vi "Left and Right Parts.vi"(0 "after":string, 1 "before":string) -> (2 "left start":string, 3 "left end":string, 4 "right start":string, 5 "right end":string)   [LabVIEW 2017, in "NI_Gmath.lvlib"]
uses:
  <vilib>/gmath/NI_Gmath.lvlib
panel:
  # "`"
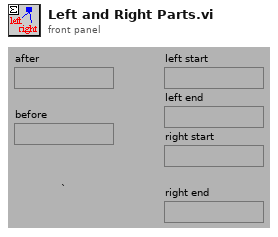
[diagram p1: front panel]
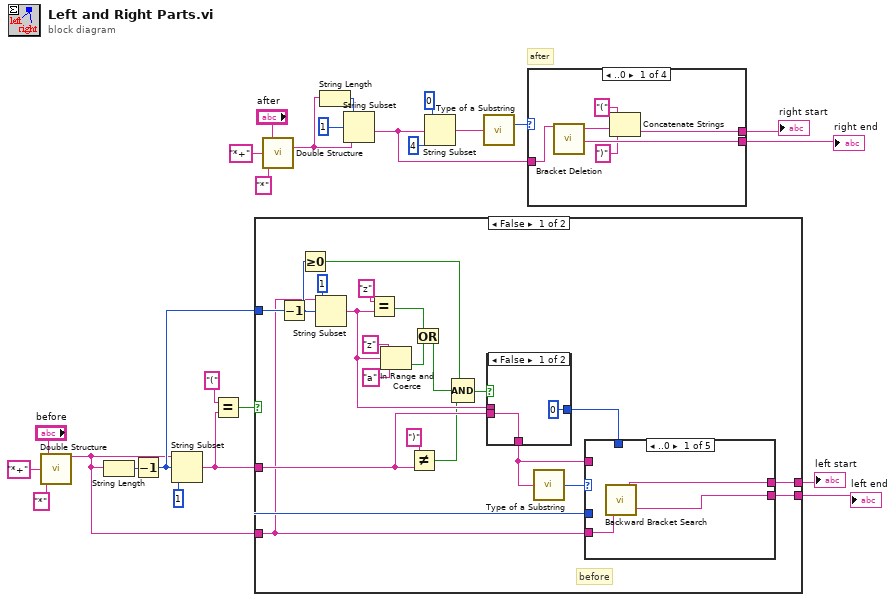
[diagram p0: block diagram]
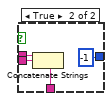
[diagram p2: hidden frame]
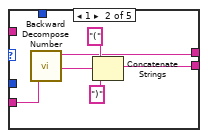
[diagram p3: hidden frame]
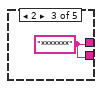
[diagram p4: hidden frame]
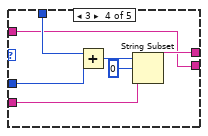
[diagram p5: hidden frame]
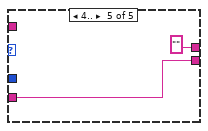
[diagram p6: hidden frame]
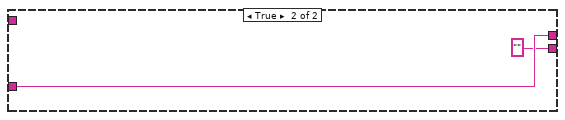
[diagram p7: hidden frame]
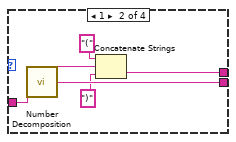
[diagram p8: hidden frame]
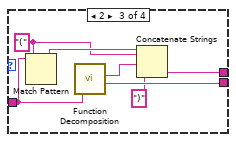
[diagram p9: hidden frame]
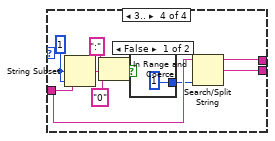
[diagram p10: hidden frame]
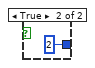
[diagram p11: hidden frame]
diagram:
  # "after"
  n1 = call <vilib>:"Double Structure.vi"("change"="*", "-+ structure"="*+", "string"="before") -> ("- structure"=w1:string)
  n2 = String Length(string=w1) -> (length=w17:i32)
  n3 = Decrement(x=w17) -> (x-1=w24:i32)
  n4 = String Subset(string=w1, offset (0)=w24, length (rest)=1) -> (substring=w16:string)
  n5 = Equal?(x="(", y=w16) -> (x = y?=w14:bool)
  n6 = case shown="False" w14 {
    tunnel: [w39 "" ("string start")] -> w10
    tunnel: [w37 w73] -> w12
    tunnel: w16 -> [w35 _]
    tunnel: w24 -> [w34 _]
    tunnel: w1 -> [w29 w73]
    frame False {
      # "before"
      n7 = Decrement(x=w34) -> (x-1=w36:i32)
      n8 = Greater Or Equal To 0?(x=w36) -> (x >= 0?=w26:bool)
      n9 = String Subset(string=w29, offset (0)=w36, length (rest)=1) -> (substring=w45:string)
      n10 = Equal?(x="z", y=w45) -> (x = y?=w27:bool)
      n11 = In Range and Coerce(upper limit="z", x=w45, lower limit="a") -> (In Range?=w40:bool)  [unwired: 1 out]
      n12 = Not Equal?(x=")", y=w35) -> (x != y?=w31:bool)
      n13 = Or(x=w27, y=w40) -> (x .or. y?=w32:bool)
      n14 = Compound Arithmetic op=AND(w26, w32, w31) -> (w33:bool)
      n15 = case shown="False" w33 {
        tunnel: w45 -> [_ w52]
        tunnel: w35 -> [w48 w51]
        tunnel: [w48 w50] -> w28
        tunnel: [0 -1] -> w38
        frame False {
        }
        frame True {
          n16 = Concatenate Strings(w52, w51) -> (w50:string)
        }
      }
      n17 = call <vilib>:"Type of a Substring.VI"("item"=w28) -> ("type"=w30:i32)
      n18 = case shown="..0" w30 {
        tunnel: w29 -> [w55 w56 _ w68 w70]
        tunnel: [w54 w57 w62 w69 ""] -> w37
        tunnel: [w53 w58 w62 w63 w70] -> w39
        tunnel: w38 -> [_ _ _ w66 _]
        tunnel: w34 -> [_ _ _ w67 _]
        tunnel: w28 -> [_ _ _ w63 _]
        frame ..0 {
          n19 = call <vilib>:"Backward Bracket Search.VI"("string input with brackets"=w55) -> ("string start"=w54:string, "string rest"=w53:string)
        }
        frame 1 {
          n20 = call <vilib>:"Backward Decompose Number.VI"("number as string"=w56) -> ("string start"=w57:string, "string rest"=w59:string)
          n21 = Concatenate Strings("(", w59, ")") -> (w58:string)
        }
        frame 2 {
          w62 = "*******"
        }
        frame 3 {
          n22 = Add(x=w66, y=w67) -> (x+y=w65:i32)
          n23 = String Subset(string=w68, offset (0)=0, length (rest)=w65) -> (substring=w69:string)
        }
        frame 4.. {
        }
      }
    }
    frame True {
    }
  }
  "left start" <- w12
  "left end" <- w10
  n24 = call <vilib>:"Double Structure.vi"("change"="*", "-+ structure"="*+", "string"="after") -> ("- structure"=w7:string)
  n25 = String Length(string=w7) -> (length=w22:i32)
  n26 = String Subset(string=w7, offset (0)=1, length (rest)=w22) -> (substring=w25:string)
  n27 = String Subset(string=w25, offset (0)=0, length (rest)=4) -> (substring=w23:string)
  n28 = call <vilib>:"Type of a Substring.VI"("item"=w23) -> ("type"=w9:i32)
  n29 = case shown="..0" w9 {
    tunnel: w25 -> [w74 w85 w91 w96]
    tunnel: [w75 w82 w88 w94] -> w13
    tunnel: [w79 w84 w92 w93] -> w11
    frame ..0 {
      n30 = call <vilib>:"Bracket Deletion.vi"("string input with brackets"=w74) -> ("string output balanced"=w76:string, "string output rest"=w79:string)  [unwired: 1 in, 1 out]
      n31 = Concatenate Strings("(", w76, ")") -> (w75:string)
    }
    frame 1 {
      n32 = call <vilib>:"Number Decomposition.VI"("number string"=w85) -> ("number"=w83:string, "rest"=w84:string)  [unwired: 1 in, 1 out]
      n33 = Concatenate Strings("(", w83, ")") -> (w82:string)
    }
    frame 2 {
      w89 = "("
      n34 = Match Pattern(string=w91, regular expression=w89) -> (before substring=w90:string)  [unwired: 1 in, 3 out]
      n35 = call <vilib>:"Function Decomposition.VI"("function string"=w91) -> ("function brackets"=w86:string, "rest"=w92:string)  [unwired: 1 in, 2 out]
      n36 = Concatenate Strings(w90, w89, w86, ")") -> (w88:string)
    }
    frame 3.. {
      w101 = 1
      n37 = String Subset(string=w96, offset (0)=w101, length (rest)=w101) -> (substring=w100:string)
      n38 = In Range and Coerce(upper limit=":", x=w100, lower limit="0") -> (In Range?=w97:bool)  [unwired: 1 out]
      n39 = case shown="False" w97 {
        tunnel: [1 2] -> w95
        frame False {
        }
        frame True {
        }
      }
      n40 = Search/Split String(string=w96, offset (0)=w95) -> (substring before match=w94:string, match + rest of string=w93:string)  [unwired: 1 in, 1 out]
    }
  }
  "right start" <- w13
  "right end" <- w11
